vi "GEvt-Set Source Filter Rules - v1.2.vi"(8 "Error In":errorcluster caption="error in (no error)", 11 "Rules-v1.2":T3) -> (0 "error out":errorcluster)   [LabVIEW 2017, in "Communicable State Machine.lvlib"]
doc: "### GEvt-Set Source Filter Rules - v1.0.vi\n\n-- <b>Controls</b> --\n- <b>Rules-v1</b>:"
uses:
  Communicable State Machine.lvlib
  Typedef/_CSM_GlobalLog_MSG_TYPE.ctl
  Typedef/_CSM_GlobalLog_STATE_TYPE.ctl
  Typedef/_CSM_GlobalLog Filter Rules - v1.2.ctl
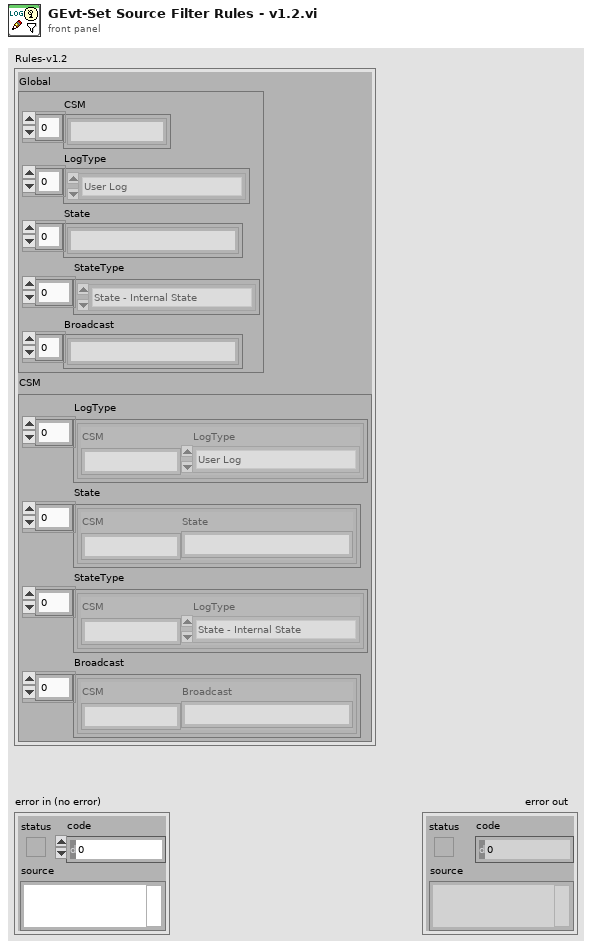
[diagram p1: front panel]
types:
  T1 = typedef "Communicable State Machine.lvlib/_CSM_GlobalLog_MSG_TYPE.ctl" = enum16{"User Log", "State Change", "Status", "Interrupt", "Register", "Unregister", "Error Log", "Module Created", "Module Destroyed", "Async Message", "No-Rep Async Message", "Sync Message", "AsyncMsg Complete", "SyncMsg Complete"}
  T2 = typedef "Communicable State Machine.lvlib/_CSM_GlobalLog_STATE_TYPE.ctl" = enum16{"State - Internal State", "State - External Message", "State - Response", "State - Complete"}
  T3 = cluster{"Global":cluster{"CSM":string[], "LogType":T1[], "State":string[], "StateType":T2[], "Broadcast":string[]}, "CSM":cluster{"LogType":cluster{"CSM":string, "LogType":T1}[], "State":cluster{"CSM":string, "State":string}[], "StateType":cluster{"CSM":string, "LogType":T2}[], "Broadcast":cluster{"CSM":string, "Broadcast":string}[]}}
  T4 = typedef "Communicable State Machine.lvlib/_CSM_GlobalLog Filter Rules - v1.2.ctl" = cluster{"Global":cluster{"CSM":string[], "LogType":T1[], "State":string[], "StateType":T2[], "Broadcast":string[]}, "CSM":cluster{"LogType":cluster{"CSM":string, "LogType":T1}[], "State":cluster{"CSM":string, "State":string}[], "StateType":cluster{"CSM":string, "LogType":T2}[], "Broadcast":cluster{"CSM":string, "Broadcast":string}[]}, "PeriodicMessageFilter":cluster{"Enable":bool, "Threshold(#/s)":dbl, "CheckPeriod(s)":dbl}}
  T5 = cluster{"CSM":string[], "LogType":T1[], "State":string[], "StateType":T2[], "Broadcast":string[]}
  T6 = cluster{"LogType":cluster{"CSM":string, "LogType":T1}[], "State":cluster{"CSM":string, "State":string}[], "StateType":cluster{"CSM":string, "LogType":T2}[], "Broadcast":cluster{"CSM":string, "Broadcast":string}[]}
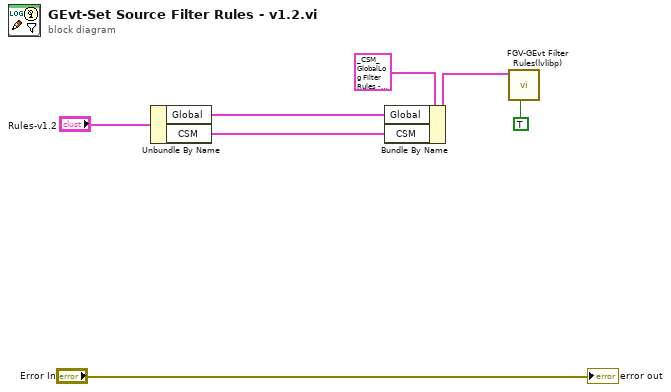
[diagram p0: block diagram]
diagram:
  n1 = Unbundle By Name("Rules-v1.2") -> ("Global"=w2:T5, "CSM"=w1:T6)
  n2 = Bundle By Name(cluster=T4 {"Global"={"CSM"=[], "LogType"=[], "State"=[], "StateType"=[], "Broadcast"=[]}, "CSM"={"LogType"=[], "State"=[], "StateType"=[], "Broadcast"=[]}, "PeriodicMessageFilter"={"Enable"=FALSE, "Threshold(#/s)"=2.0, "CheckPeriod(s)"=1.0}} ("Rules-v1.2"), "Global"=w2, "CSM"=w1) -> (w4:T4)
  n3 = call "FGV-GEvt Filter Rules(lvlibp).vi"("Set? (T)/Get(F)"=TRUE ("Set(T)/Get(F)"), "Rules-v1.2"=w4) -> ()  [unwired: 8 in, 2 out]
  "error out" <- "Error In"
